vi "IPI_ReadLaserValue.vi"(8 "错误输入（无错误）":errorcluster, 11 "VISA资源名称":refnum<visa-resource-name>) -> (0 "错误输出":errorcluster, 2 "LaserValue":string, 3 "VISA资源名称输出":refnum<visa-resource-name>, 5 "读取缓冲区":string)   [LabVIEW 2015]
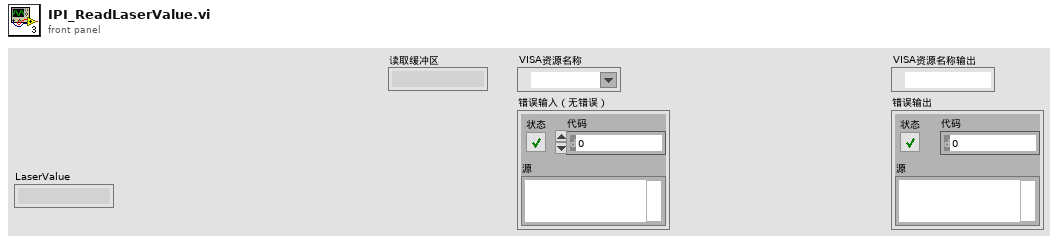
[diagram p1: front panel]
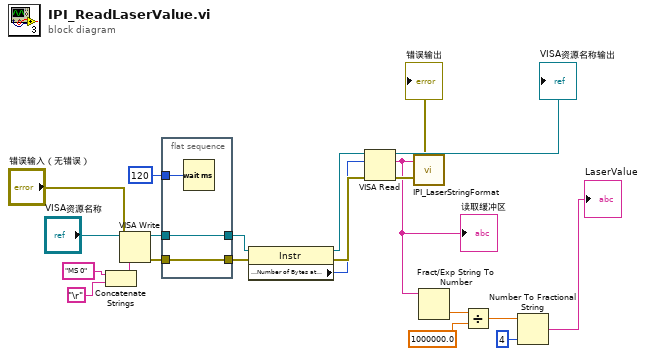
[diagram p0: block diagram]
diagram:
  n1 = Concatenate Strings("MS 0" ("Command"), "\r") -> (w14:string)
  n2 = VISA Write(VISA resource name="VISA资源名称", write buffer=w14, error in (no error)="错误输入（无错误）") -> (VISA resource name out=w19:refnum<visa-resource-name>, error out=w21:errorcluster)  [unwired: 1 out]
  n3 = flat-sequence {
    tunnel: w21 -> [w23]
    tunnel: [w23] -> w20
    tunnel: w19 -> [w22]
    tunnel: [w22] -> w18
    tunnel: u32 120 ("读取前延时(ms)") -> [w24]
    frame #0 {
      n4 = Wait (ms)(milliseconds to wait=w24) -> ()  [unwired: 1 out]
    }
  }
  n5 = property class="Instr"(reference=w18, error in=w20) -> (reference out=w17:refnum<visa-resource-name>, error out=w16:errorcluster, "Serial Settings:Number of Bytes at Serial Port"=w15:u32)
  n6 = VISA Read(VISA resource name=w17, byte count=w15, error in (no error)=w16) -> (VISA resource name out=→"VISA资源名称输出":refnum<visa-resource-name>, read buffer=w6:string, error out=→"错误输出":errorcluster)  [unwired: 1 out]
  "读取缓冲区" <- w6
  n7 = call "IPI_LaserStringFormat.vi"("响应"=w6) -> ()  [unwired: 9 in, 2 out]
  n8 = Fract/Exp String To Number(string=w6) -> (number=w5:dbl)  [unwired: 3 in, 1 out]
  n9 = Divide(x=w5, y=1000000.0) -> (x/y=w3:dbl)
  n10 = Number To Fractional String(number=w3, precision (6)=i16 4 ("精度(6)")) -> (F-format string=→"LaserValue":string)  [unwired: 2 in]
